vi "Vision Processing For Cool People.vi"(4 "Range":cluster{"Lower value":sgl, "Upper value":sgl}={"Lower value"=234.67392, "Upper value"=255.0} {"Lower value" scale=0.0..255.0; "Upper value" scale=0.0..255.0}, 5 "Image Size":T2, 6 "View 2":bool, 7 "Original Image":T3(plugin-control)) -> (0 "Target Found?":bool, 1 "Processed Image":T3(plugin-control), 2 "Position":cluster{"X":dbl, "Y":dbl}, 3 "Target Info":T1(array[cluster]))   [LabVIEW 2011]
uses:
  <vilib>/Rock Robotics/WPI/Camera/WPI_CameraImageSize.ctl
  <vilib>/vision/NI_Vision_Development_Module.lvlib
panel:
  in  "4":bool
  in  "3":bool
  in  "2":bool
  in  "1":bool
  in  "Processing":enum32{"Color", "Intensity", "Intensity Open"}(tab)=enum."Intensity"
  in  "Luminance":i32=255
  in  "Saturation":i32=255
  in  "Hue":i32(knob)=65 scale=0.0..255.0
  in  "Margins":cluster{"Hue":i32, "Sat":i32, "Lum":i32}={"Hue"=20, "Sat"=27, "Lum"=30} {"Sat" scale=0.0..40.0; "Lum" scale=0.0..40.0; "Hue" scale=0.0..40.0}
  in  "Range 2":cluster{"Lower value":sgl, "Upper value":sgl}={"Lower value"=234.67392, "Upper value"=255.0} {"Lower value" scale=0.0..255.0; "Upper value" scale=0.0..255.0}
  in  "Particle Count Limit":i32=8
  in  "Area Size Limit":i32=444
  in  "Score Limits":T4={"Rect Coverage"=76.0, "Aspect Ratio"=70.0, "X Edge Strength"=40.0, "Y Edge Strength"=60.0}
  in  "Camera Type":enum16{"206", "1011"}(ring)=enum."1011"
  in  "View":bool
  out "Original Image 2":T3(plugin-control)
  # "This SubVI gets a camera picture from the Dashboard, marks rectangular shapes and finds their\nDistance (in inches or meters).\nColor Processing finds the target by it's color. However, should the target be lighted with any sort of flashlight\npointing roughly at the same direction as the Camera's lens, it's easier to use Intensity Processing as the rectangular targets\nare Retro-Reflective and it's very easy to distinguish their intensity."
  # "Camera type affects:\n1. Extracting a single plane from a color image (useful for Intensity Processing) \n2. Camera's view angle for distance calculation."
  # "Note: the X and Y values are measured from the target's center.\nDistance is measured from the camera's lens to the target's center."
  # "That's the indicator of the original image."
  # "That's the control the SubVI receives as an input."
  # "That's the processed image."
  # "RECOMMENDED\nLower value: 234\nUpper value: 255\nConsidering the retro-reflective target is lighted"
  # "RECOMMENDED\nLower value: 234\nUpper value: 255\nConsidering the retro-reflective target is lighted"
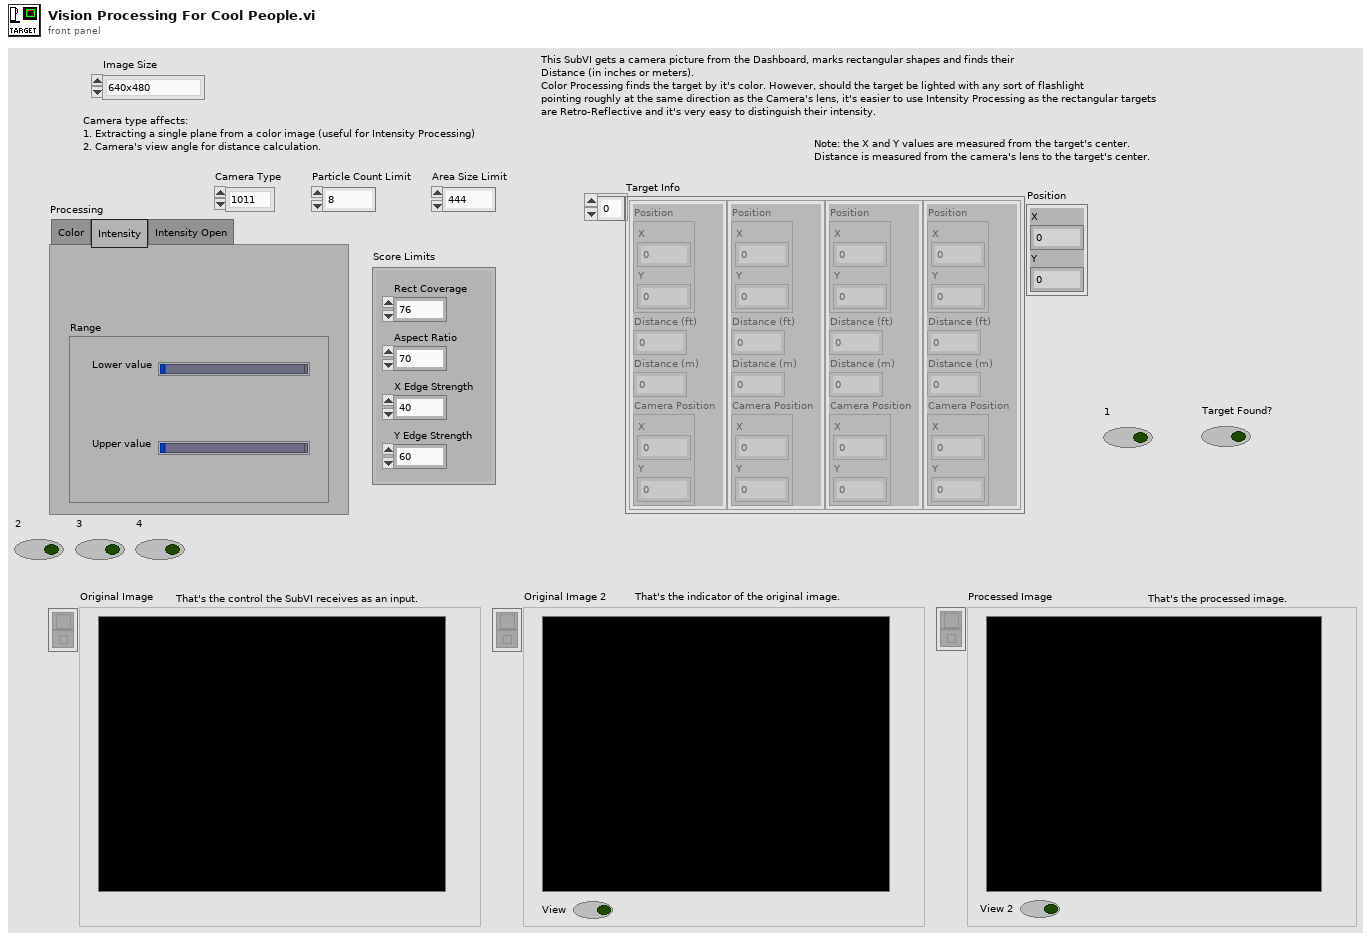
[diagram p1: front panel]
types:
  T1 = cluster{"Position":cluster{"X":dbl, "Y":dbl}, "Distance (ft)":dbl, "Distance (m)":dbl, "Camera Position":cluster{"X":dbl, "Y":dbl}}[]
  T2 = typedef "WPI_CameraImageSize.ctl" = enum16{"640x480", "320x240", "160x120"}
  T3 = typedef "IMAQ Image.ctl" = refnum<image>
  T4 = cluster{"Rect Coverage":dbl, "Aspect Ratio":dbl, "X Edge Strength":dbl, "Y Edge Strength":dbl}
  T5 = typedef "Image Type" = u32
  T6 = enum32{"AutoM", "Close", "Dilate", "Erode", "Gradient", "Gradient out", "Gradient in", "Hit miss", "Open", "PClose", "POpen", "Thick", "Thin"}
  T7 = cluster{cluster{"Left":dbl, "Top":dbl, "Right":dbl, "Bottom":dbl}, dbl[]}[]
  T8 = cluster{"Left":dbl, "Top":dbl, "Right":dbl, "Bottom":dbl}
  T9 = cluster{"Target Center (-1 to 1)":cluster{"X":dbl, "Y":dbl}, "Distance (ft)":dbl, "Distance (m)":dbl, "Target Center (Camera)":cluster{"X":dbl, "Y":dbl}}
  T10 = cluster{"Target Center (-1 to 1)":cluster{"X":dbl, "Y":dbl}, "Distance (ft)":dbl, "Distance (m)":dbl, "Target Center (Camera)":cluster{"X":dbl, "Y":dbl}}[]
  T11 = cluster{"Position":cluster{"X":dbl, "Y":dbl}, "Distance (ft)":dbl, "Distance (m)":dbl, "Camera Position":cluster{"X":dbl, "Y":dbl}}
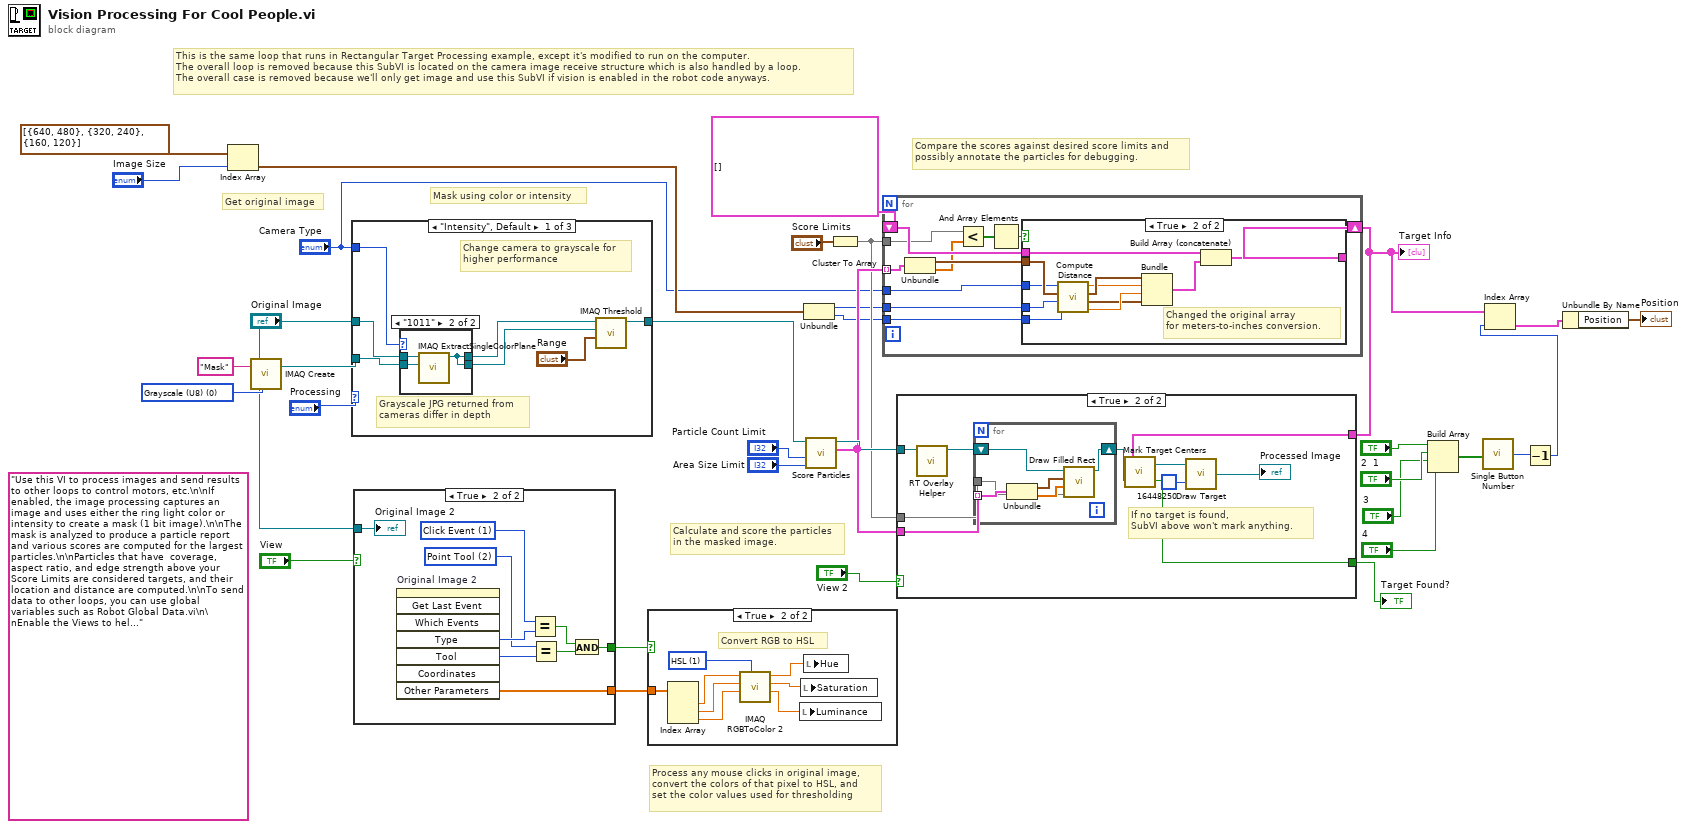
[diagram p0: block diagram]
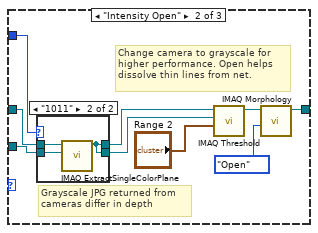
[diagram p4: hidden frame]
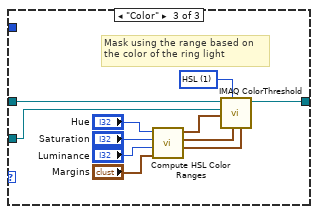
[diagram p6: hidden frame]
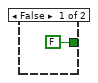
[diagram p7: hidden frame]
diagram:
  w34 = T5 0 items=["Grayscale (U8)", "Grayscale (I16)", "Grayscale (SGL)", "Complex (CSG)", "RGB (U32)", "HSL (U32)", "RGB (U64)", "Grayscale (U16)"] ("Image Type")
  (unwired) "Use this VI to process images and send results to other loops to control motors, etc.\n\nIf enabled, the image processing captures an image and uses either the ring light color or intensity to create a mask (1 bit image).\n\nThe mask is analyzed to produce a particle report and various scores are computed for the largest particles.\n\nParticles that have  coverage, aspect ratio, and edge strength above your Score Limits are considered targets, and their location and distance are computed.\n\nTo send data to other loops, you can use global variables such as Robot Global Data.vi\n\nEnable the Views to help debug color settings. Disable the View to speed up processing."
  # "Compare the scores against desired score limits and\npossibly annotate the particles for debugging."
  # "Process any mouse clicks in original image,\nconvert the colors of that pixel to HSL, and\nset the color values used for thresholding"
  # "Calculate and score the particles\nin the masked image."
  # "Mask using color or intensity"
  # "Get original image"
  # "This is the same loop that runs in Rectangular Target Processing example, except it's modified to run on the computer.\nThe overall loop is removed because this SubVI is located on the camera image receive structure which is also handled by a loop.\nThe overall case is removed because we'll only get image and use this SubVI if vision is enabled in the robot code anyways."
  n1 = Index Array(array=cluster{i32, i32}[] [{640, 480}, {320, 240}, {160, 120}], index="Image Size") -> (element=w14:cluster{i32, i32})
  n2 = call "IMAQ Create"("Image Name"="Mask", "Image Type"=w34) -> ("New Image"=w32:T3)  [unwired: 2 in, 2 out]
  n3 = case shown="\"Intensity\", Default" "Processing" {
    tunnel: "Original Image" -> [w39 w49 w71]
    tunnel: [w40 w52 w70] -> w19
    tunnel: w32 -> [w38 w50 w61]
    tunnel: "Camera Type" -> [w37 w51 _]
    frame "Intensity", Default {
      # "Grayscale JPG returned from\ncameras differ in depth"
      # "Change camera to grayscale for\nhigher performance"
      n4 = case shown="\"1011\"" w37 {
        tunnel: w39 -> [w43 w46]
        tunnel: w38 -> [w42 w45]
        tunnel: [w43 w44] -> w36
        tunnel: [w42 w44] -> w35
        frame "206", Default {
        }
        frame "1011" {
          n5 = call "IMAQ ExtractSingleColorPlane"("Image Dst"=w45, "Image Src"=w46) -> ("Image Dst Out"=w44:T3)  [unwired: 8 in, 1 out]
        }
      }
      n6 = call "IMAQ Threshold"("Range"="Range", "Image Dst"=w35, "Image Src"=w36) -> ("Image Dst Out"=w40:T3)  [unwired: 3 in, 5 out]
    }
    frame "Intensity Open" {
      # "Grayscale JPG returned from\ncameras differ in depth"
      # "Change camera to grayscale for\nhigher performance. Open helps\ndissolve thin lines from net."
      n7 = case shown="\"1011\"" w51 {
        tunnel: w49 -> [w57 w60]
        tunnel: w50 -> [w56 w59]
        tunnel: [w57 w58] -> w48
        tunnel: [w56 w58] -> w47
        frame "206", Default {
        }
        frame "1011" {
          n8 = call "IMAQ ExtractSingleColorPlane"("Image Dst"=w59, "Image Src"=w60) -> ("Image Dst Out"=w58:T3)  [unwired: 8 in, 1 out]
        }
      }
      n9 = call "IMAQ Threshold"("Range"="Range 2", "Image Dst"=w47, "Image Src"=w48) -> ("Image Dst Out"=w53:T3)  [unwired: 3 in, 5 out]
      n10 = call "IMAQ Morphology"("Operation"=T6."Open", "Image Src"=w53) -> ("Image Dst Out"=w52:T3)  [unwired: 8 in, 1 out]
    }
    frame "Color" {
      w69 = u16 1 items=["RGB", "HSL", "HSV", "HSI"] ("Color Mode")
      # "Mask using the range based on\nthe color of the ring light"
      n11 = call "Compute HSL Color Ranges.vi"("Margins"="Margins", "Luminance"="Luminance", "Saturation"="Saturation", "Hue"="Hue") -> ("Lum Range"=w66:cluster{i32, i32}, "Sat Range"=w67:cluster{i32, i32}, "Hue Range"=w68:cluster{i32, i32})  [unwired: 5 in]
      n12 = call "IMAQ ColorThreshold"("Blue or Luma or Val or Inten Range"=w66, "Green or Sat Range"=w67, "Color Mode"=w69, "Red or Hue Range"=w68, "Image Dst"=w61, "Image Src"=w71) -> ("Image Dst Out"=w70:T3)  [unwired: 4 in, 1 out]
    }
  }
  n13 = case shown="True" "View" {
    tunnel: "Original Image" -> [_ w80]
    tunnel: [_ w75] -> w18
    tunnel: [_ w72] -> w17
    frame False {
    }
    frame True {
      w73 = 2 items=["None", "Selection Tool", "Point Tool", "Line Tool", "Rectangle Tool", "Oval Tool", "Polygon Tool", "ClosedFreehandTool", "Annulus Tool", "Rotated Rectangle Tool", "Zoom Tool", "Pan Tool", "Polyline Tool", "Freehand Tool"] ("Tool")
      w74 = 1 items=["No Event"=0, "Click Event"=1, "Draw Event"=2, "Size Event"=4, "Scroll Event"=5, "Double Click Event"=8] ("Type")
      n14 = invoke on="Original Image 2" class="ImageControl" method="Get Last Event"() -> ("Type"=w76:i32, "Tool"=w79:i32, "Other Parameters"=w72:sgl[])  [unwired: 8 in, 5 out]
      n15 = Equal?(x=w74, y=w76) -> (x = y?=w77:bool)
      n16 = Equal?(x=w73, y=w79) -> (x = y?=w78:bool)
      n17 = And(x=w77, y=w78) -> (x .and. y?=w75:bool)
      "Original Image 2" <- w80
    }
  }
  n18 = case shown="True" w18 {
    tunnel: w17 -> [_ w88]
    frame False {
    }
    frame True {
      w87 = u16 1 items=["RGB", "HSL", "HSV", "HSI", "CIE L*a*b*", "CIE XYZ"] ("Color Mode")
      # "Convert RGB to HSL"
      n19 = Index Array(array=w88) -> (element #1=w86:sgl, element #2=w84:sgl, element #3=w82:sgl)  [unwired: 3 in]
      n20 = call "IMAQ RGBToColor 2"("Color Mode"=w87, "Blue value"=w82, "Green value"=w84, "Red value"=w86) -> ("Blue or Luma or Val or Inten or Z or b*value"=w81:dbl, "Green or Sat or Y or a* value"=w83:dbl, "Red or Hue or X or L* value"=w85:dbl)  [unwired: 4 in, 1 out]
      n21 = local write "Luminance"(w81) -> ()
      n22 = local write "Saturation"(w83) -> ()
      n23 = local write "Hue"(w85) -> ()
    }
  }
  n24 = Unbundle(w14) -> (w16:i32, w15:i32)
  n25 = call "Score Particles.vi"("Area Size Limit"="Area Size Limit", "Particle Count Limit"="Particle Count Limit", "Image Refnum in"=w19) -> ("Scored Particle Info"=w25:T7, "Image Refnum out"=w28:T3)  [unwired: 7 in]
  n26 = Cluster To Array(cluster="Score Limits") -> (array=w23:dbl[])
  n27 = for {
    shift-right: [w98] -> w5
    shift-left: T1 [] -> [w99]
    tunnel: w16 -> [w97]
    tunnel: w25 -> [w95] mode=indexing
    tunnel: w23 -> [w90]
    tunnel: "Camera Type" -> [w94]
    tunnel: w15 -> [w89]
    n28 = Unbundle(w95) -> (w96:T8, w91:dbl[])
    n29 = Less?(x=w90, y=w91) -> (x < y?=w93:bool[])
    n30 = And Array Elements(Boolean array=w93) -> (logical AND=w92:bool)
    n31 = case shown="True" w92 {
      tunnel: w99 -> [w100 w111]
      tunnel: [w100 w101] -> w98
      tunnel: w96 -> [_ w109]
      tunnel: w97 -> [_ w110]
      tunnel: w94 -> [_ w108]
      tunnel: w89 -> [_ w107]
      frame False {
      }
      frame True {
        # "Changed the original array\nfor meters-to-inches conversion."
        n32 = call "Compute Distance.vi"("Y Image Resolution"=w107, "X Image Resolution"=w110, "Bounding Box"=w109, "Camera Type"=w108) -> ("Distance (m)"=w103:dbl, "Target Center (Camera)"=w102:cluster{"X":dbl, "Y":dbl}, "Target Center (-1 to 1)"=w105:cluster{"X":dbl, "Y":dbl}, "Distance (ft)"=w104:dbl)  [unwired: 4 in]
        n33 = Bundle("Target Center (-1 to 1)"=w105, "Distance (ft)"=w104, "Distance (m)"=w103, "Target Center (Camera)"=w102) -> (w106:T9)  [unwired: 1 in]
        n34 = Build Array (concatenate)(w111, w106) -> (w101:T10)
      }
    }
  }
  "Target Info" <- w5
  n35 = case shown="True" "View 2" {
    tunnel: w28 -> [_ w119]
    tunnel: w25 -> [_ w121]
    tunnel: w23 -> [_ w120]
    tunnel: w5 -> [_ w117]
    tunnel: [FALSE ("Target") w113] -> w1
    frame False {
    }
    frame True {
      # "If no target is found,\nSubVI above won't mark anything."
      n36 = call "RT Overlay Helper.vi"("Refnum in"=w119) -> ("Refnum out"=w122:T3)  [unwired: 10 in]
      n37 = for {
        shift-right: [w127] -> w118
        shift-left: w122 -> [w128]
        tunnel: w121 -> [w124] mode=indexing
        tunnel: w120 -> [w123]
        n38 = Unbundle(w124) -> (w125:T8, w126:dbl[])
        n39 = call "Draw Filled Rect.vi"("Limits"=w123, "Scores"=w126, "Bounding Box"=w125, "image in"=w128) -> ("image out"=w127:T3)  [unwired: 7 in]
      }
      n40 = call "Mark Target Centers.vi"("Processed Image"=w118, "Target Info"=w117) -> ("Target"=w113:bool, "Image Out"=w116:T3)
      n41 = call "Draw Target.vi"("Color"=u32 16448250, "Original Image"=w116) -> ("Image Out"=→"Processed Image":T3)
    }
  }
  "Target Found?" <- w1
  n42 = Build Array("1", "2", "3", "4") -> (w7:bool[])
  n43 = call "Single Button Number.vi"("Bool Array"=w7) -> ("Number"=w6:i32)
  n44 = Decrement(x=w6) -> (x-1=w4:i32)
  n45 = Index Array(array=w5, index=w4) -> (element=w3:T11)
  n46 = Unbundle By Name(w3) -> ("Position"=→"Position":cluster{"X":dbl, "Y":dbl})
